vi "Bachelor's Thesis.vi"() -> ()   [LabVIEW 2025]
uses:
  <vilib>/DAQmx/read.llb/DAQmx Read (Analog 2D DBL NChan NSamp).vi
  <vilib>/MakerHub/LINX/Public/Peripherals/PWM/PWM Set Duty Cycle 1 Chan.vi
  <vilib>/MakerHub/LINX/Public/Utilities/Open Serial.vi
  <vilib>/DAQmx/create/channels.llb/DAQmx Create Channel (AI-Voltage-Basic).vi
  <vilib>/DAQmx/configure/timing.llb/DAQmx Timing (Sample Clock).vi
  <vilib>/DAQmx/miscellaneous.llb/DAQmx Fill In Error Info.vi
  <vilib>/measure/mascope.llb/Pulse Measurements 1 chan.vi
  <vilib>/addons/control/pid/pid.llb/PID (DBL).vi
  <vilib>/MakerHub/LINX/Public/Peripherals/PWM/PWM Set Duty Cycle N Chans.vi
  <vilib>/MakerHub/LINX/LMH-LINX.lvlib
  <vilib>/addons/control/pid/NI_PID_pid.lvlib
  <vilib>/measure/NI_MAPro.lvlib
panel:
  out "V_total":dbl
  out "Result":string
  out "Curent circuit":dbl format="%#_3g"
  in  "Rezistenta de referinta":dbl=330.0
  out "Tensiunea R":dbl format="%#_3g"
  in  "Test":path
  out "Culoare LED detectatã":string
  out "Tensiune prag LED":dbl format="%#_3g"
  out "Waveform Graph":dbl[](graph)
  out "Waveform Chart":cluster{"Duty cycle":dbl, "upper limit":dbl}(graph)
  in  "PID gains":T1={"proportional gain (Kc)"=1.0, "integral time (Ti, min)"=0.01, "derivative time (Td, min)"=0.0} {"derivative time (Td, min)" format="%.3f"; "integral time (Ti, min)" format="%.3f"; "proportional gain (Kc)" format="%.3f"}
  in  "Duty cycle":dbl(slide) scale=0.0..1.0
  out "LED":dbl(slide) scale=0.0..1.0
  in  "stop":bool
  # "V"
  # "mA"
  # "V"
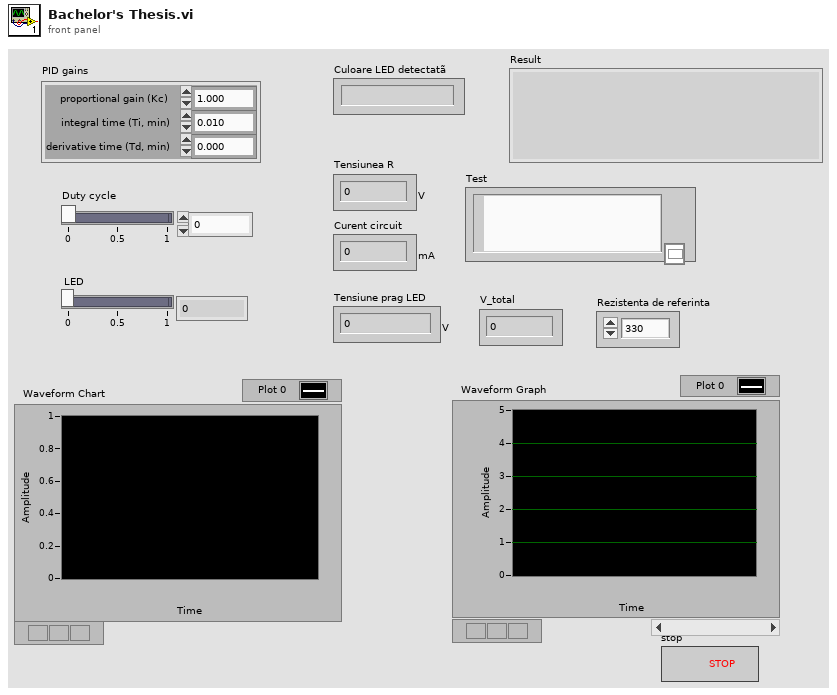
[diagram p1: front panel]
types:
  T1 = cluster{"proportional gain (Kc)":dbl, "integral time (Ti, min)":dbl, "derivative time (Td, min)":dbl}
  T2 = typedef "LMH-LINX.lvlib/LINX Ref.ctl" = cluster{"IO":T3, "Interface":T4, "LINX Device Config":T5}
  T3 = typedef "LMH-LINX.lvlib/Platform.ctl" = enum16{"Remote", "Local"}
  T4 = typedef "LMH-LINX.lvlib/Interface.ctl" = enum16{"Serial", "TCP"}
  T5 = typedef "LMH-LINX.lvlib/Device.lvlib/LINX Device Config.ctl" = cluster{"Interface":T4, "COM Port":refnum<visa-resource-name>, "TCP Configuration":T6, "Device Family":u8, "Device ID":u8, "Device Name":string, "TCP Ref":refnum<k5>, "Channels":T7}
  T6 = typedef "LMH-LINX.lvlib/Device.lvlib/TCP Config.ctl" = cluster{"IP Address":string, "Port":u16}
  T7 = typedef "LMH-LINX.lvlib/Channels.ctl" = cluster{"DI":u8[], "DO":u8[], "AI":u8[], "AO":u8[], "PWM":u8[], "QE":u8[], "UART":u8[], "I2C 2":u8[], "SPI":u8[], "CAN":u8[], "Servo":u8[], "AI Ref (V)":dbl, "AI Resolution (Bits)":u8, "AO Ref (V)":dbl, "AO Resolution (Bits)":u8}
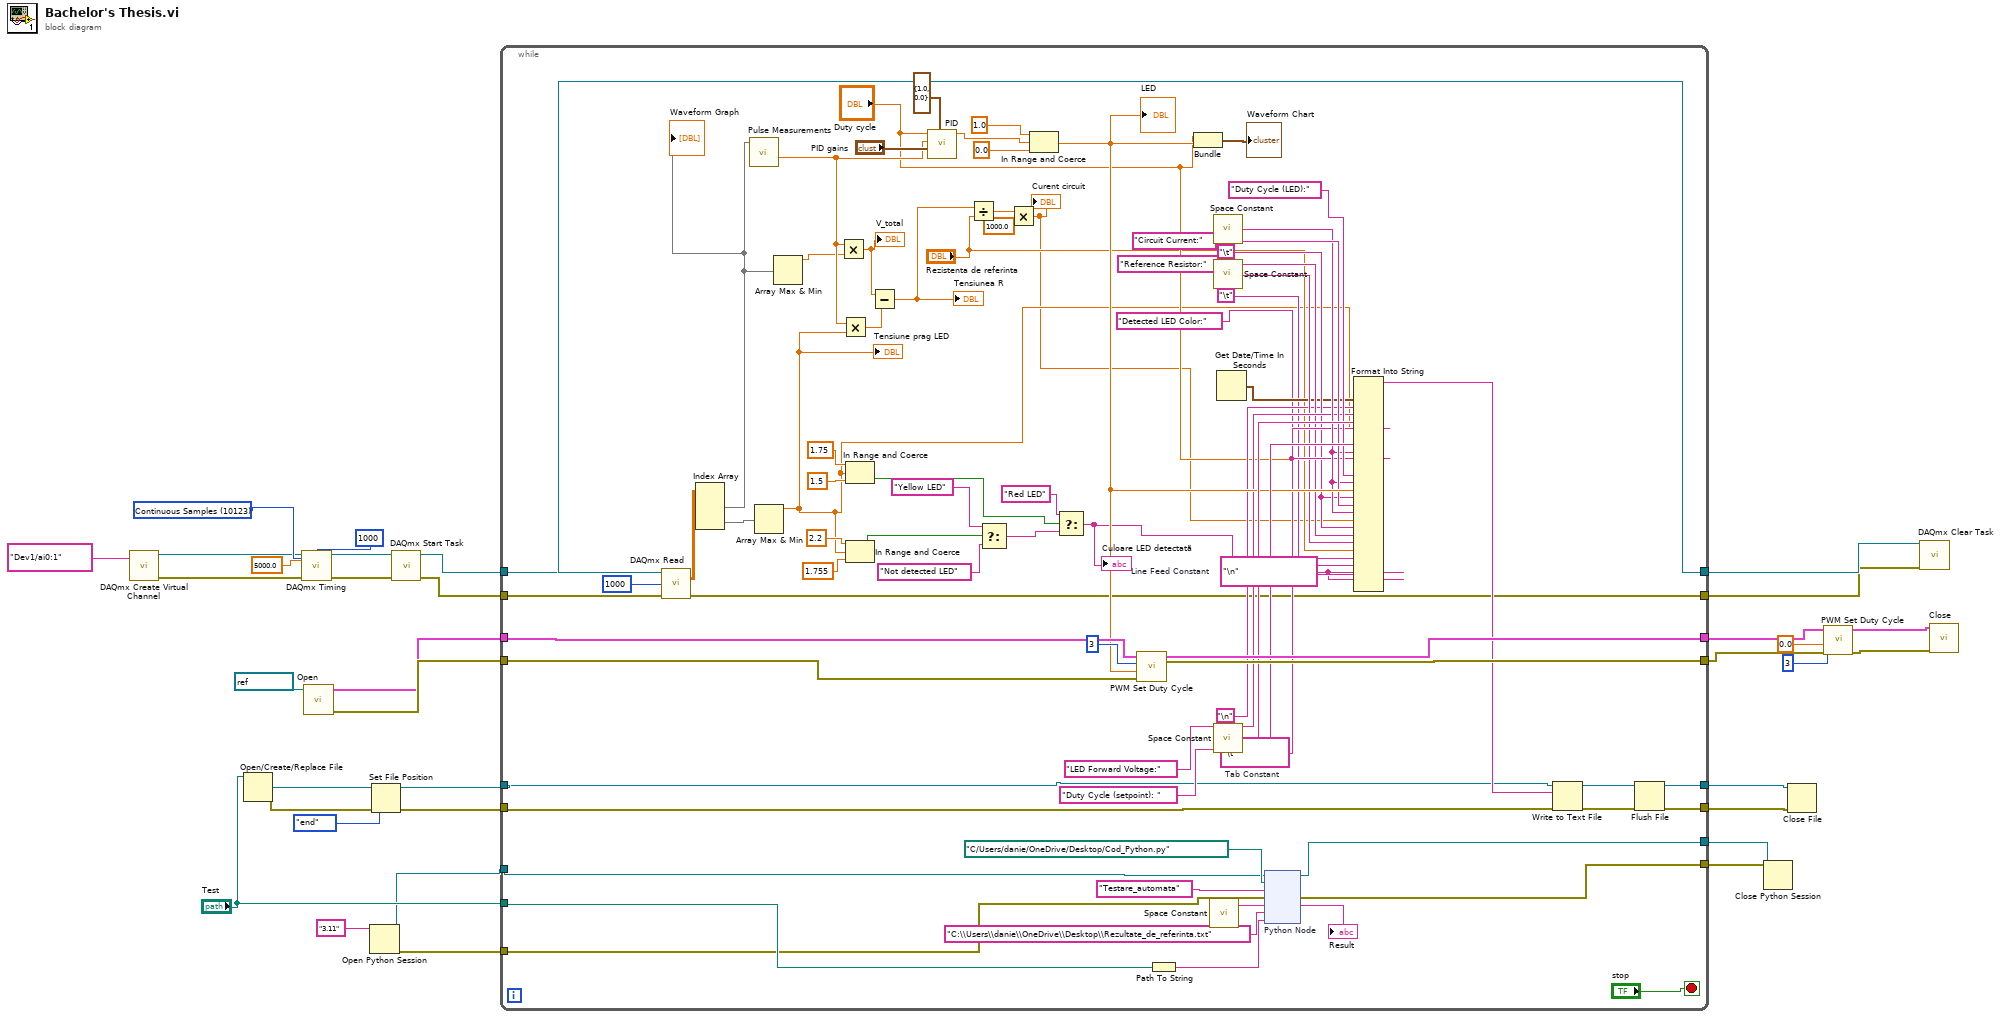
[diagram p0: block diagram]
diagram:
  w28 = 10123 items=["Finite Samples"=10178, "Continuous Samples"=10123, "Hardware Timed Single Point"=12522] ("sample mode")
  n1 = call-poly <vilib>:"DAQmx Create Virtual Channel.vi"("physical channels"=tag "Dev1/ai0:1") -> ("task out"=w20:refnum<k21>, "error out"=w19:errorcluster)  [unwired: 13 in]
  n2 = Open/Create/Replace File(file path (use dialog)="Test") -> (refnum out=w12:refnum<file>, error out=w11:errorcluster)  [unwired: 5 in, 1 out]
  n3 = call-poly <vilib>:"DAQmx Timing.vi"("task/channels in"=w20, "sample mode"=w28, "samples per channel"=1000, "rate"=5000.0, "error in"=w19) -> ("task out"=w25:refnum<k21>, "error out"=w24:errorcluster)  [unwired: 9 in]
  n4 = call-poly <vilib>:"Open.vi"("Serial Port"=refnum<visa-resource-name> "COM3") -> ("Error Out"=w34:errorcluster, "LINX Resource"=w33:T2)  [unwired: 8 in, 1 out]
  n5 = Open Python Session(python version="3.11" ("Python version")) -> (session out=w16:refnum<k35>, error out=w7:errorcluster)  [unwired: 2 in]
  n6 = Set File Position(refnum=w12, from (0:start)=enum16{"start", "end", "current"}."end", error in=w11) -> (refnum out=w9:refnum<file>, error out=w10:errorcluster)  [unwired: 1 in]
  n7 = call <vilib>:"DAQmx Start Task.vi"("task/channels in"=w25, "error in"=w24) -> ("task out"=w23:refnum<k21>, "error out"=w22:errorcluster)  [unwired: 12 in]
  n8 = while {
    tunnel: w33 -> [w109]
    tunnel: [w108] -> w6
    tunnel: w34 -> [w110]
    tunnel: [w107] -> w5
    tunnel: [w104] -> w30
    tunnel: [w56] -> w26
    tunnel: w23 -> [w99]
    tunnel: w22 -> [w98]
    tunnel: "Test" -> [w49]
    tunnel: w16 -> [w45]
    tunnel: [w44] -> w14
    tunnel: [w43] -> w13
    tunnel: w9 -> [w55]
    tunnel: [w40] -> w18
    tunnel: w10 -> [w80]
    tunnel: [w39] -> w21
    tunnel: w7 -> [w36]
    stop <- "stop" stop-if-true
    w63 = "\n"  # Line Feed Constant
    w71 = "\t"
    w73 = "\t"  # Tab Constant
    n9 = call-poly <vilib>:"DAQmx Read.vi"("task/channels in"=w99, "number of samples per channel"=1000, "error in"=w98) -> ("task out"=w104:refnum<k21>, "data"=w96:dbl[][], "error out"=w56:errorcluster)  [unwired: 10 in]
    n10 = Index Array "Index Array"(array=w96) -> (element #1=w95:dbl[], element #2=w94:dbl[])  [unwired: 4 in]
    "Waveform Graph" <- w95
    n11 = call-poly <vilib>:"Pulse Measurements.vi"("signal in"=w95) -> ("duty cycle"=w93:dbl)  [unwired: 6 in, 4 out]
    n12 = Array Max & Min(array=w94) -> (max value=w53:dbl)  [unwired: 3 out]
    "Tensiune prag LED" <- w53
    n13 = Array Max & Min(array=w95) -> (max value=w61:dbl)  [unwired: 3 out]
    n14 = Multiply(x=w93, y=w61) -> (x*y=w92:dbl)
    "V_total" <- w92
    n15 = Multiply(x=w93, y=w53) -> (x*y=w54:dbl)
    n16 = In Range and Coerce(upper limit=1.75, x=w53, lower limit=1.5) -> (In Range?=w89:bool)  [unwired: 1 out]
    n17 = In Range and Coerce(upper limit=2.2, x=w53, lower limit=1.755) -> (In Range?=w85:bool)  [unwired: 1 out]
    n18 = Subtract(x=w92, y=w54) -> (x-y=w60:dbl)
    "Tensiunea R" <- w60
    n19 = call-poly <vilib>:"PID.vi"("output range"=cluster{"output high":dbl, "output low":dbl} {"output high"=1.0, "output low"=0.0}, "PID gains"="PID gains", "process variable"=w93, "setpoint"="Duty cycle") -> ("output"=w103:dbl)  [unwired: 6 in, 1 out]
    n20 = Divide(x=w60, y="Rezistenta de referinta") -> (x/y=w58:dbl)
    n21 = Select(t="Yellow LED", s=w85, f="Not detected LED") -> (s? t:f=w82:string)
    n22 = Multiply(x=w58, y=1000.0) -> (x*y=w52:dbl)
    "Curent circuit" <- w52
    n23 = In Range and Coerce(upper limit=1.0, x=w103, lower limit=0.0) -> (coerced(x)=w76:dbl)  [unwired: 1 out]
    "LED" <- w76
    n24 = Select(t="Red LED", s=w89, f=w82) -> (s? t:f=w64:string)
    "Culoare LED detectatã" <- w64
    n25 = call-poly <vilib>:"PWM Set Duty Cycle.vi"("Error In"=w110, "Duty Cycle (0-1)"=w76, "PWM Channel"=u8 3, "LINX Resource"=w109) -> ("Error Out"=w107:errorcluster, "LINX Resource"=w108:T2)  [unwired: 6 in]
    n26 = Path To String(path=w49) -> (string=w51:string)
    n27 = Bundle "Bundle"("Duty cycle"="Duty cycle", "upper limit"=w76) -> (→"Waveform Chart":cluster{"Duty cycle":dbl, "upper limit":dbl})  [unwired: 1 in]
    n28 = call <vilib>:"Space Constant.vi"() -> ("String"=w37:string)
    n29 = call <vilib>:"Space Constant.vi"() -> ("String"=w74:string)
    n30 = call <vilib>:"Space Constant.vi"() -> ("String"=w69:string)
    n31 = call <vilib>:"Space Constant.vi"() -> ("String"=w79:string)
    n32 = Get Date/Time In Seconds() -> (seconds since 1Jan1904=w68:timestamp)
    n33 = node "Python Node"(w45, path "C:/Users/danie/OneDrive/Desktop/Cod_Python.py" ("module path"), "Testare_automata" ("function name"), w36, w37, "C:\\Users\\danie\\OneDrive\\Desktop\\Rezultate_de_referinta.txt", w51) -> (w44:refnum<k35>, w43:errorcluster, →"Result":string)  [unwired: 2 in, 2 out]
    n34 = Format Into String "Format Into String"(w68, "\n", "LED Forward Voltage:" ("initial string"), w79, w53, w73, "Duty Cycle (setpoint): " ("input 6"), w74, "Duty cycle", w73, "Duty Cycle (LED):" ("input 6"), w74, w76, w71, "Circuit Current:" ("input 6"), w74, w52, w71, "Reference Resistor:" ("input 6"), w69, "Rezistenta de referinta", "\t", "Detected LED Color:" ("input 6"), w64, w63, w63) -> (resulting string=w81:string)  [unwired: 3 in, 1 out]
    n35 = Write to Text File(file (use dialog)=w55, text=w81, error in=w80) -> (refnum out=w42:refnum<file>, error out=w41:errorcluster)  [unwired: 1 in, 1 out]
    n36 = Flush File(refnum=w42, error in=w41) -> (refnum out=w40:refnum<file>, error out=w39:errorcluster)
  }
  n37 = Close Python Session(session in=w14, error in=w13) -> ()  [unwired: 1 out]
  n38 = Close File(refnum=w18, error in=w21) -> ()  [unwired: 2 out]
  n39 = call-poly <vilib>:"PWM Set Duty Cycle.vi"("Error In"=w5, "Duty Cycle (0-1)"=0.0, "PWM Channel"=u8 3, "LINX Resource"=w6) -> ("Error Out"=w2:errorcluster, "LINX Resource"=w1:T2)  [unwired: 6 in]
  n40 = call <vilib>:"DAQmx Clear Task.vi"("task in"=w30, "error in"=w26) -> ()  [unwired: 13 in, 1 out]
  n41 = call <vilib>:"Close.vi"("Error In"=w2, "LINX Resource"=w1) -> ()  [unwired: 9 in, 1 out]
